vi "time.vi"(8 "Error In":errorcluster) -> (0 "Error Out":errorcluster, 1 "only date":string, 2 "datetime":string, 3 "date/time string":string, 5 "current time":timestamp)   [LabVIEW 2023]
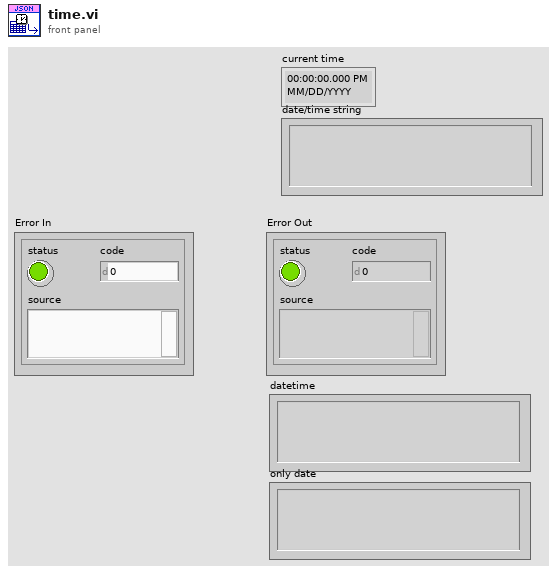
[diagram p1: front panel]
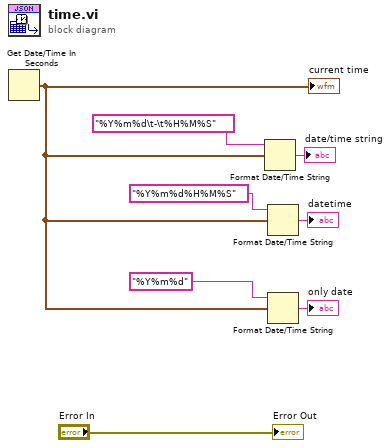
[diagram p0: block diagram]
diagram:
  n1 = Get Date/Time In Seconds() -> (seconds since 1Jan1904=w1:timestamp)
  "current time" <- w1
  n2 = Format Date/Time String(time format string (%c)="%Y%m%d\t-\t%H%M%S", seconds (now)=w1) -> (date/time string=→"date/time string":string)  [unwired: 1 in]
  n3 = Format Date/Time String(time format string (%c)="%Y%m%d%H%M%S", seconds (now)=w1) -> (date/time string=→"datetime":string)  [unwired: 1 in]
  n4 = Format Date/Time String(time format string (%c)="%Y%m%d", seconds (now)=w1) -> (date/time string=→"only date":string)  [unwired: 1 in]
  "Error Out" <- "Error In"
